vi "Update UserInfo In Panel.vi"(8 "error in (no error)":errorcluster, 10 "UI Ref":refnum<vi>[](array[refnum]), 11 "MemberInfo in":refnum<class "Information.lvclass">) -> (0 "error out":errorcluster, 2 "UserInfo":T1, 3 "MemberInfo out":refnum<class "Information.lvclass">)   [LabVIEW 2015, in "Information.lvclass"]
uses:
  Information.lvclass
  Type Definitions/UserInfo.ctl
  Information.lvclass/Information.ctl
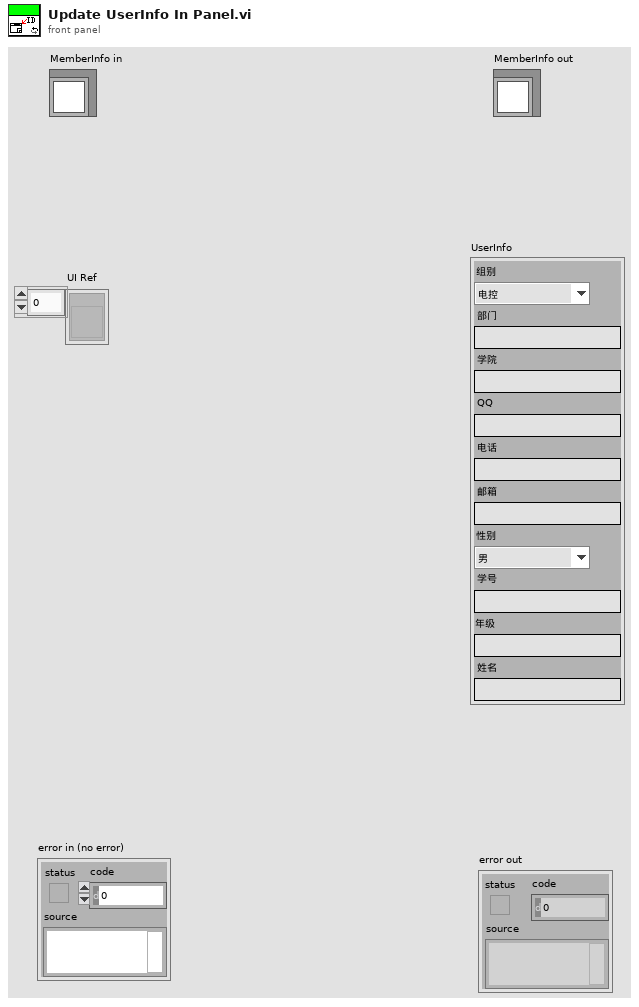
[diagram p1: front panel]
types:
  T1 = typedef "Information.lvclass/UserInfo.ctl" = cluster{"组别":enum16{"电控", "机械", "视觉"}, "部门":string, "学院":string, "QQ":string, "电话":string, "邮箱":string, "性别":enum16{"男", "女"}, "学号":string, "年级":string, "姓名":string}
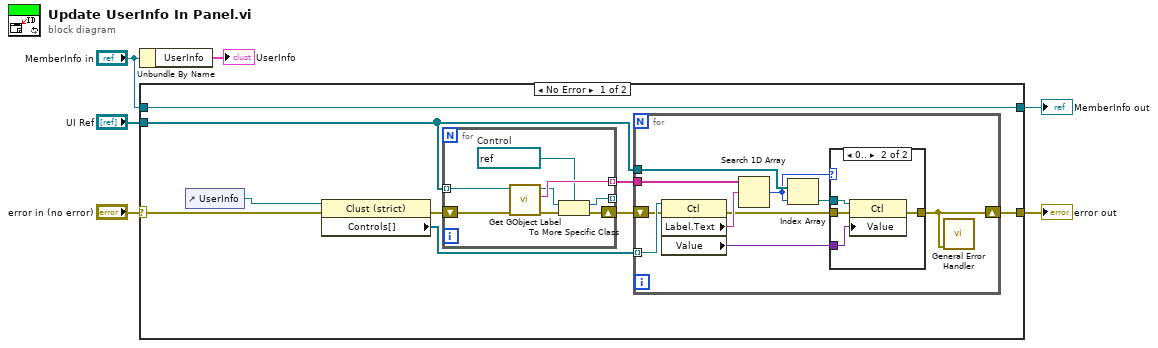
[diagram p0: block diagram]
diagram:
  n1 = Unbundle By Name("MemberInfo in") -> ("UserInfo"=→"UserInfo":T1)
  n2 = case shown="No Error" "error in (no error)" {
    selector: "error in (no error)" -> [w10 w40]
    tunnel: [w11 w40] -> w5
    tunnel: [w15 w39] -> w4
    tunnel: "MemberInfo in" -> [w15 w39]
    tunnel: "UI Ref" -> [w9 _]
    frame No Error {
      n3 = control-ref of="UserInfo"() -> (w7:refnum<vi>)
      n4 = property class="Clust (strict)"(reference=w7, error in=w10) -> (error out=w8:errorcluster, "Controls[]"=w14:refnum<vi>[])  [unwired: 1 out]
      n5 = for {
        tunnel: w9 -> [w21] mode=indexing
        shift-right: [w16] -> w13
        shift-left: w8 -> [w22]
        tunnel: [w17] -> _ mode=indexing
        tunnel: [w23] -> w12 mode=indexing
        w20 = refnum<vi> refnum  # Control
        n6 = call <vilib>:"Get GObject Label.vi"("error in (no error)"=w22, "GObject"=w21) -> ("error out"=w19:errorcluster, "Object Label"=w23:string, "dup GObject"=w18:refnum<vi>)  [unwired: 5 in, 2 out]
        n7 = To More Specific Class(target class=w20, reference=w18, error in=w19) -> (specific class reference=w17:refnum<vi>, error out=w16:errorcluster)
      }
      n8 = for {
        tunnel: w14 -> [w33] mode=indexing
        tunnel: w9 -> [w29]
        tunnel: w12 -> [w31]
        shift-right: [w28] -> w11
        shift-left: w13 -> [w32]
        n9 = property class="Ctl"(reference=w33, error in=w32) -> (error out=w25:errorcluster, "Label.Text"=w30:string, "Value"=w26:variant)  [unwired: 1 out]
        n10 = Search 1D Array(1D array=w31, element=w30) -> (index of element=w24:i32)  [unwired: 1 in]
        n11 = Index Array(array=w29, index=w24) -> (element=w27:refnum<vi>)
        n12 = case shown="0.." w24 {
          tunnel: [w34 w38] -> w28
          tunnel: w27 -> [_ w37]
          tunnel: w26 -> [_ w36]
          tunnel: w25 -> [w34 w35]
          frame Default {
          }
          frame 0.. {
            n13 = property class="Ctl"(reference=w37, error in=w35, "Value"=w36) -> (error out=w38:errorcluster)  [unwired: 1 out]
          }
        }
        n14 = call <vilib>:"General Error Handler.vi"("error in (no error)"=w28) -> ()  [unwired: 10 in, 5 out]
      }
    }
    frame Error {
    }
  }
  "error out" <- w5
  "MemberInfo out" <- w4
